vi "google search.vi"() -> ()   [LabVIEW 2018]
panel:
  in  "stop":bool
  in  "String":string
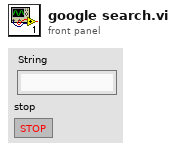
[diagram p1: front panel]
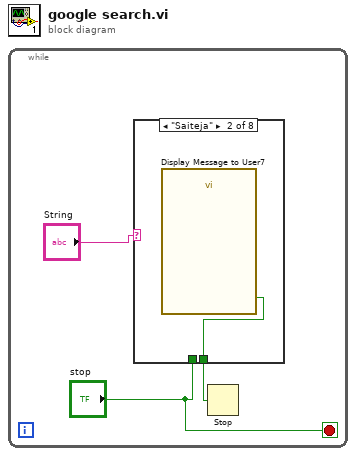
[diagram p0: block diagram]
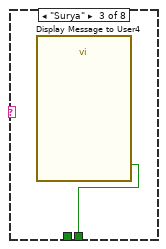
[diagram p3: hidden frame]
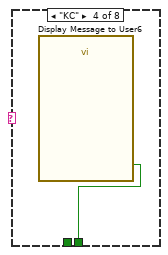
[diagram p4: hidden frame]
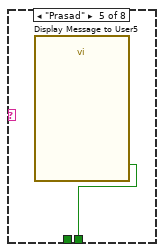
[diagram p5: hidden frame]
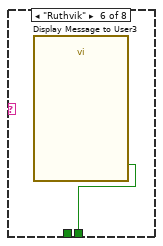
[diagram p6: hidden frame]
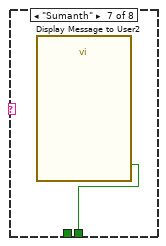
[diagram p7: hidden frame]
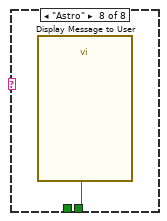
[diagram p8: hidden frame]
diagram:
  n1 = while {
    stop <- "stop" stop-if-true
    n2 = case shown="\"Saiteja\"" "String" {
      tunnel: [w4 w5 w6 w7 w8 w9 w10 w11] -> w2
      tunnel: "stop" -> [w4 _ _ _ _ _ _ _]
      frame "False", Default {
      }
      frame "Saiteja" {
        n3 = call "Display Message to User7"() -> ("OK"=w5:bool)  [unwired: 10 in, 1 out]
      }
      frame "Surya" {
        n4 = call "Display Message to User4"() -> ("OK"=w6:bool)  [unwired: 10 in, 1 out]
      }
      frame "KC" {
        n5 = call "Display Message to User6"() -> ("OK"=w7:bool)  [unwired: 10 in, 1 out]
      }
      frame "Prasad" {
        n6 = call "Display Message to User5"() -> ("OK"=w8:bool)  [unwired: 10 in, 1 out]
      }
      frame "Ruthvik" {
        n7 = call "Display Message to User3"() -> ("OK"=w9:bool)  [unwired: 10 in, 1 out]
      }
      frame "Sumanth" {
        n8 = call "Display Message to User2"() -> ("OK"=w10:bool)  [unwired: 10 in, 1 out]
      }
      frame "Astro" {
        n9 = call "Display Message to User"() -> ("OK"=w11:bool)  [unwired: 10 in, 1 out]
      }
    }
    n10 = Stop(stop? (T)=w2) -> ()
  }
